vi "xy图绘制圆.vi"() -> ()   [LabVIEW 2025]
panel:
  in  "红圆的半径":dbl
  in  "白圆的半径":dbl
  out "XY图 2":cluster{dbl[], dbl[]}[](graph)
  out "XY图":cluster{dbl[], dbl[]}(graph)
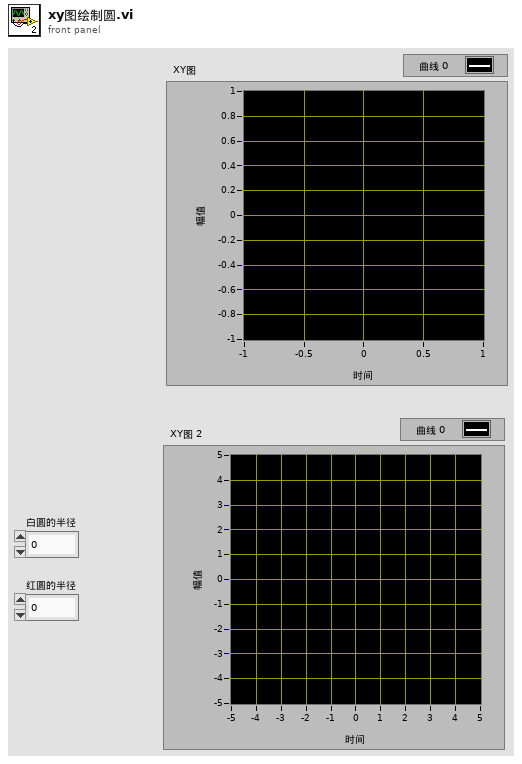
[diagram p1: front panel]
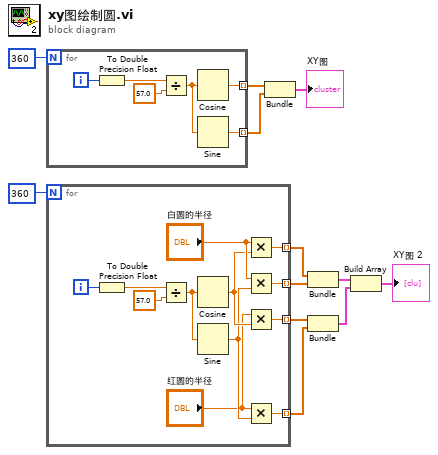
[diagram p0: block diagram]
diagram:
  n1 = for {
    N: 360 -> [_]
    tunnel: [w15] -> w11 mode=indexing
    tunnel: [w13] -> w9 mode=indexing
    i -> [w16]
    n2 = To Double Precision Float(number=w16) -> (double precision float=w17:dbl)
    n3 = Divide(x=w17, y=57.0) -> (x/y=w14:dbl)
    n4 = Cosine(x=w14) -> (cos(x)=w13:dbl)
    n5 = Sine(x=w14) -> (sin(x)=w15:dbl)
  }
  n6 = for {
    N: 360 -> [_]
    tunnel: [w24] -> w7 mode=indexing
    tunnel: [w26] -> w6 mode=indexing
    tunnel: [w20] -> w3 mode=indexing
    tunnel: [w19] -> w2 mode=indexing
    i -> [w28]
    n7 = To Double Precision Float(number=w28) -> (double precision float=w29:dbl)
    n8 = Divide(x=w29, y=57.0) -> (x/y=w27:dbl)
    n9 = Cosine(x=w27) -> (cos(x)=w23:dbl)
    n10 = Sine(x=w27) -> (sin(x)=w22:dbl)
    n11 = Multiply(x="白圆的半径", y=w23) -> (x*y=w26:dbl)
    n12 = Multiply(x="白圆的半径", y=w22) -> (x*y=w24:dbl)
    n13 = Multiply(x="红圆的半径", y=w23) -> (x*y=w20:dbl)
    n14 = Multiply(x="红圆的半径", y=w22) -> (x*y=w19:dbl)
  }
  n15 = Bundle(w9, w11) -> (→"XY图":cluster{dbl[], dbl[]})  [unwired: 1 in]
  n16 = Bundle(w6, w7) -> (w5:cluster{dbl[], dbl[]})  [unwired: 1 in]
  n17 = Bundle(w3, w2) -> (w1:cluster{dbl[], dbl[]})  [unwired: 1 in]
  n18 = Build Array(w5, w1) -> (→"XY图 2":cluster{dbl[], dbl[]}[])
